vi "Queue Array Destroy.vi"(8 "error in (no error)":errorcluster, 11 "queue name in":string[](array[string])) -> (0 "error out":errorcluster, 3 "queue name out":string[](array[string]))   [LabVIEW 2020]
uses:
  Control/Queue Data.ctl
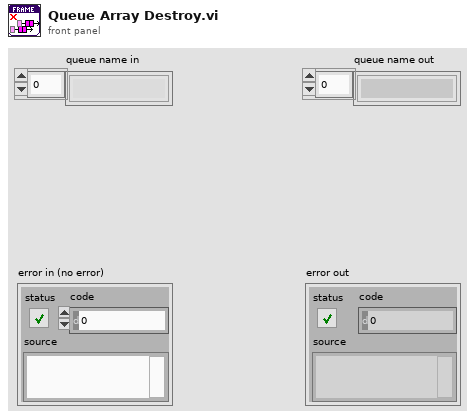
[diagram p1: front panel]
types:
  T1 = typedef "Queue Data.ctl" = cluster{"event":string, "data":variant}
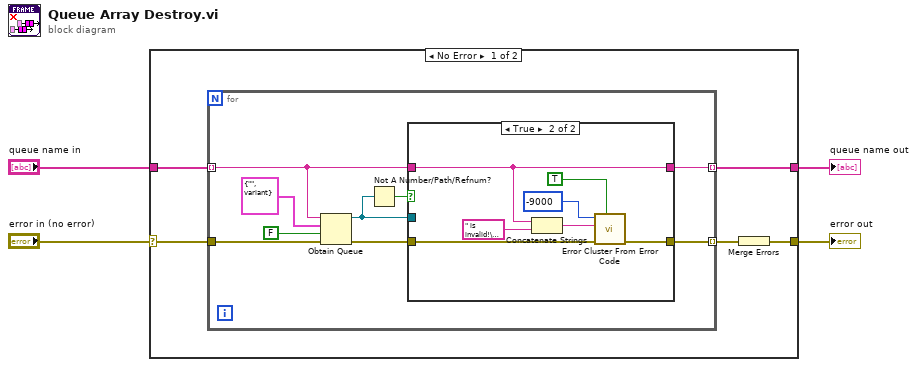
[diagram p0: block diagram]
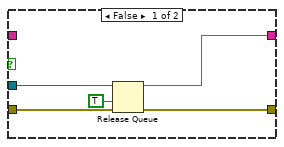
[diagram p2: hidden frame]
diagram:
  n1 = case shown="No Error" "error in (no error)" {
    selector: "error in (no error)" -> [w7 w32]
    tunnel: [w5 w32] -> w3
    tunnel: "queue name in" -> [w9 w31]
    tunnel: [w8 w31] -> w1
    frame No Error {
      n2 = for {
        tunnel: w9 -> [w13] mode=indexing
        tunnel: [w12] -> w8 mode=indexing
        tunnel: w7 -> [w11]
        tunnel: [w10] -> w6 mode=indexing
        n3 = Obtain Queue(name (unnamed)=w13, element data type=T1 {"event"="", "data"=variant}, create if not found? (T)=FALSE, error in (no error)=w11) -> (queue out=w15:refnum<queue>, error out=w16:errorcluster)  [unwired: 1 in, 1 out]
        n4 = Not A Number/Path/Refnum?(number/path/refnum=w15) -> (NaN/Path/Refnum?=w14:bool)
        n5 = case shown="True" w14 {
          tunnel: w16 -> [w23 w26]
          tunnel: w15 -> [w21 _]
          tunnel: w13 -> [_ w25]
          tunnel: [w19 w25] -> w12
          tunnel: [w20 w24] -> w10
          frame False {
            n6 = Release Queue(queue=w21, force destroy? (F)=TRUE, error in (no error)=w23) -> (queue name=w19:string, error out=w20:errorcluster)  [unwired: 1 out]
          }
          frame True {
            n7 = Concatenate Strings(w25, " is invalid!\nEnsure the queue has been created!" ("字符串")) -> (w30:string)
            n8 = call <vilib>:"Error Cluster From Error Code.vi"("show call chain? (False)"=TRUE, "error in (no error)"=w26, "error message (\"\")"=w30, "error code (0)"=-9000) -> ("error out"=w24:errorcluster)  [unwired: 5 in]
          }
        }
      }
      n9 = Merge Errors(w6) -> (w5:errorcluster)
    }
    frame Error {
    }
  }
  "error out" <- w3
  "queue name out" <- w1
